vi "Flock_Logger_Process.vi"(11 "Process":string) -> ()   [LabVIEW 2013, in "Logger.lvlib"]
doc: "This asynchronous VI is launched by the Central Process. It receives status and error messages and logs them to C:\\FlockLog.txt. It will shutdown when it recieves an exit command from the Central Process."
uses:
  Logger.lvlib
  Shared Code/AMC/VI Source/LocalProcessMessaging/Flock_Shared_LocalProcessMessaging.lvlib
  Shared Code/AMC/VI Source/CentralProcessMessaging/Flock_Shared_CentralProcessMessaging.lvlib
  Shared Code/AMC/VI Source/Error Handling/Flock_ErrorHandling.lvlib
panel:
  out "Debug Status Message Value":string
  out "error out":errorcluster
  in  "error in (no error)":errorcluster
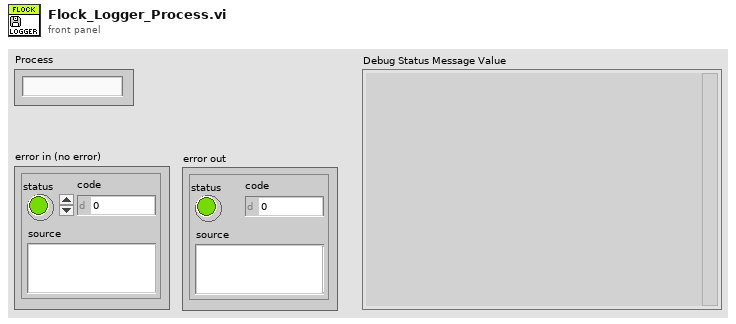
[diagram p1: front panel]
types:
  T1 = typedef "Flock_Shared_Messaging.lvlib/ProcessList.ctl" = string
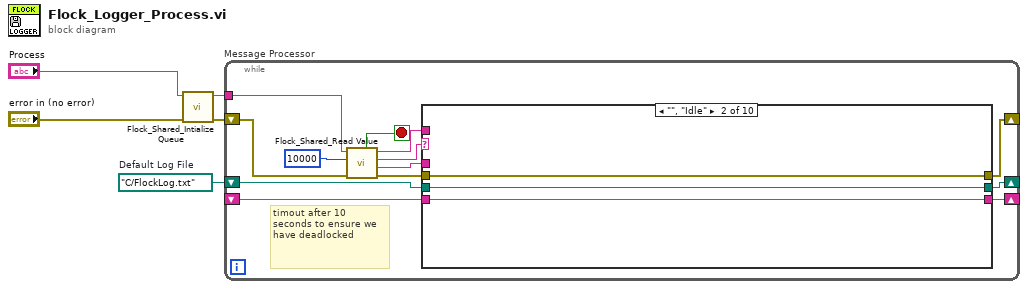
[diagram p0: block diagram]
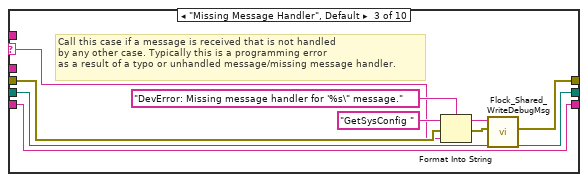
[diagram p3: hidden frame]
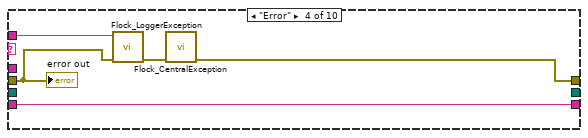
[diagram p4: hidden frame]
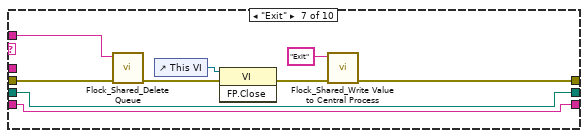
[diagram p7: hidden frame]
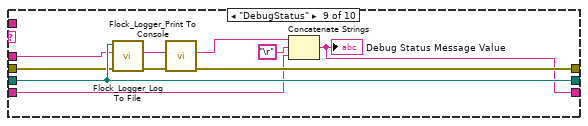
[diagram p9: hidden frame]
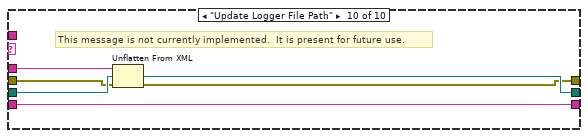
[diagram p10: hidden frame]
diagram:
  w3 = path "C:/FlockLog.txt"  # Default Log File
  n1 = call "Flock_Shared_Intialize Queue.vi"("error in (no error)"="error in (no error)", "Enum"="Process") -> ("error out"=w5:errorcluster, "Process Name"=w2:T1)  [unwired: 8 in]
  n2 = while "Message Processor" {
    shift-left: w5 -> [w18]
    shift-right: [w9] -> _
    tunnel: w2 -> [w14]
    shift-right: [w11] -> _
    shift-left: w3 -> [w12]
    shift-right: [w6] -> _
    shift-left: _ -> [w7]
    stop <- w8 stop-if-true
    # "timout after 10 seconds to ensure we have deadlocked"
    n3 = call "Flock_Shared_Read Value.vi"("error in (no error)"=w18, "timeout (1ms)"=10000, "Process"=w14) -> ("error out"=w16:errorcluster, "Message Value"=w13:string, "Message Name"=w17:string, "Process"=w10:T1, "Exit Process"=w8:bool)  [unwired: 4 in]
    n4 = case shown="\"\", \"Idle\"" w17 {
      selector: w17 -> [_ _ w26 _ _ _ _ _ _ _]
      tunnel: w16 -> [w20 w23 w27 w36 w39 w42 w47 w53 w62 w67]
      tunnel: [w20 w23 w25 w34 w39 w42 w44 w53 w60 w65] -> w9
      tunnel: w13 -> [_ _ _ _ _ _ _ _ w59 w68]
      tunnel: w12 -> [_ w22 w32 _ _ w41 w50 _ w63 w69]
      tunnel: [_ w22 w32 _ _ w41 w50 _ w63 w66] -> w11
      tunnel: w10 -> [_ _ _ w33 _ _ w51 _ _ _]
      tunnel: w7 -> [w19 w21 w24 w37 w38 w40 w48 w52 w55 w64]
      tunnel: [w19 w21 w24 w37 w38 w40 w48 w52 w54 w64] -> w6
      frame "---------- Framework Operations ----------" {
        # "Dummy case to add a seperator in the Case Structure menu"
      }
      frame "", "Idle" {
      }
      frame "Missing Message Handler", Default {
        # "Call this case if a message is received that is not handled \nby any other case. Typically this is a programming error\nas a result of a typo or unhandled message/missing message handler."
        n5 = Format Into String(format string="DevError: Missing message handler for '%s\" message." ("message"), initial string="GetSysConfig ", error in=w27, w26) -> (resulting string=w29:string, error out=w28:errorcluster)
        n6 = call "Flock_Shared_WriteDebugMsg.vi"("error in (no error)"=w28, "Current Message Case"=w29) -> ("error out"=w25:errorcluster)  [unwired: 9 in]
      }
      frame "Error" {
        n7 = call "Flock_LoggerException.vi"("Error In"=w36, "Process List"=w33) -> ("Error Out"=w35:errorcluster)  [unwired: 9 in]
        n8 = call "Flock_CentralException.vi"("Error In"=w35) -> ("Error Out"=w34:errorcluster)  [unwired: 10 in]
        "error out" <- w36
      }
      frame "---------- Generic Operations ----------" {
        # "Dummy case to add a seperator in the Case Structure menu"
      }
      frame "Initialize" {
      }
      frame "Exit" {
        n9 = call "Flock_Shared_Delete Queue.vi"("Error In"=w47, "Process Name"=w51) -> ("Error Out"=w46:errorcluster)  [unwired: 9 in]
        n10 = control-ref of="This VI"() -> (w49:refnum<vi>)
        n11 = invoke class="VI" method="FP.Close"(reference=w49, error in=w46) -> (error out=w45:errorcluster)  [unwired: 1 in, 2 out]
        n12 = call "Flock_Shared_Write Value to Central Process.vi"("error in (no error)"=w45, "Message Name"="Exit") -> ("error out"=w44:errorcluster)  [unwired: 9 in]
      }
      frame "---------- Application Operations ----------" {
      }
      frame "DebugStatus" {
        n13 = call "Flock_Logger_Log To File.vi"("error in"=w62, "Text"=w59, "File"=w63) -> ("error out"=w61:errorcluster, "TextOut"=w58:string)  [unwired: 7 in]
        n14 = call "Flock_Logger_Print To Console.vi"("Error In"=w61, "Text"=w58) -> ("Error Out"=w60:errorcluster, "TextOut"=w57:string)  [unwired: 8 in]
        n15 = Concatenate Strings(w57, "\r", w55) -> (w54:string)
        "Debug Status Message Value" <- w54
      }
      frame "Update Logger File Path" {
        # "This message is not currently implemented.  It is present for future use."
        n16 = Unflatten From XML(xml string=w68, type=w69, error in (no error)=w67) -> (value=w66:path, error out=w65:errorcluster)
      }
    }
  }
